vi "Process Injection Event Data.vi"(8 "error in (no error)":errorcluster, 10 "Injection.Results":T1 {"Measurements"."Shots"."Results"."Off-Stage Min Volt" format="%#.6g"; "Measurements"."Shots"."Results"."Off-Stage Avg Volt" format="%#.6g"; "Measurements"."Shots"."Results"."Off-Stage Max Volt" format="%#.6g"; "Measurements"."Shots"."Results"."Total Stage Time (us)" format="%#.6g"; "Measurements"."Shots"."Results"."Off-Stage Avg Current" format="%#.6g"; "Measurements"."Shots"."Results"."Total Voltage Pulses" format="%#.6g"; "Measurements"."Shots"."Results"."Off-Stage Min Current" format="%#.6g"; "Measurements"."Shots"."Results"."Off-Stage Max Current" format="%#.6g"}, 11 "Parameters":T4) -> (0 "error out":errorcluster, 3 "Parameters":T4)   [LabVIEW 2019, in "Fuel Injector Analysis Addon Engine.lvlib"]
uses:
  Fuel Injector Analysis Addon Engine.lvlib
  Types/Async Parameters.ctl
  Addon Shared/Types/Shot.Parameters.ctl
  Addon Shared/Types/Stage.Parameters.ctl
  Addon Shared/Types/Stage.PullIn.Types.ctl
  Addon Shared/Types/Stage.Transition.Types.ctl
  Addon Shared/Types/Analysis.Channels.Select.ctl
  Addon Shared/Types/Injector info.ctl
  Types/Injector.State.ctl
  <vilib>/NI/NIVS Inline Async API/_Data Access Engine/Data Access Engine/Types/Write.DVR.ctl
  <vilib>/NI/NIVS Inline Async API/_Data Access Engine/Access Type Classes/Write/Write.lvclass
  <vilib>/NI/NIVS Inline Async API/_Data Access Engine/Data Access Engine/Types/Read.DVR.ctl
  <vilib>/NI/NIVS Inline Async API/_Data Access Engine/Access Type Classes/Read/Read.lvclass
  Addon Shared/Types/Compiled.Group.WaveformRefs.ctl
  <vilib>/NI VeriStand/Custom Device API/Waveform Data Reference.ctl
  <vilib>/NI VeriStand/Custom Device Waveform API/Single Waveform Write (DBL)/Single Waveform Write (DBL).lvclass
  C:/Program Files (x86)/National Instruments/LabVIEW 2019/vi.lib/NI VeriStand/Custom Device Waveform API/Waveform Session.lvclass
  Types/Injector Event Data Cluster.ctl
  Types/Shot Information Control.ctl
  Types/Stage.Measurements.ctl
  <vilib>/NI/NIVS Inline Async API/_Data Access Engine/Access Type Classes/Read/Read.lvclass/Read.ctl
  <vilib>/NI VeriStand/Custom Device Waveform API/Waveform Session.lvclass/Waveform Session.ctl
  <vilib>/NI VeriStand/Custom Device Waveform API/Single Waveform Write (DBL)/Single Waveform Write (DBL).lvclass/Single Waveform Write (DBL).ctl
  <vilib>/NI VeriStand/Custom Device Waveform API/Internal Comm Classes/WPL Comm/WPL Comm (1D DBL)/WPL Comm (1D DBL).lvclass/WPL Comm (1D DBL).ctl
  <vilib>/NI VeriStand/Custom Device Waveform API/Internal Comm Classes/WPL Comm/WPL Comm.lvclass/WPL Comm.ctl
  <vilib>/NI/NIVS Inline Async API/_Data Access Engine/Access Type Classes/Write/Write.lvclass/Write.ctl
  <vilib>/NI VeriStand/Custom Device Waveform API/NI VeriStand - Write Waveform(s).vi
  <vilib>/NI VeriStand/Custom Device Waveform API/Single Waveform Write (DBL)/NI VeriStand - Write Single Waveform (DBL).vi
  <vilib>/NI/NIVS Inline Async API/_Data Access Engine/Data Access Engine/Methods/Data.Processes.Execute.vi
  <vilib>/NI/NIVS Inline Async API/_Data Access Engine/Data Access Engine/Methods/Read.Data.vi
  Build Result Array from Shots.vi
  <vilib>/NI/NIVS Inline Async API/_Data Access Engine/Data Access Engine/Methods/Write.Data.vi
  Calculate Current Magnitude Measurements.vi
  RT.Stages.Find.vi
  <vilib>/NI VeriStand/Custom Device Waveform API/Internal Comm Classes/WPL Comm/WPL Comm (1D DBL)/Comm_write 1d dbl.vi
  <vilib>/NI VeriStand/Custom Device Waveform API/Read Sample offset DVR.vi
  <vilib>/NI VeriStand/Custom Device Waveform API/Check Opened.vi
  <vilib>/NI/NIVS Inline Async API/_Data Access Engine/Access Type Classes/Read/Read.ProcessData.vi
  <vilib>/NI/NIVS Inline Async API/_Data Access Engine/Access Type Classes/Write/Write.ProcessData.vi
  Calculate Hold-In Measurements.vi
  <vilib>/Analysis/baseanly.llb/Mean.vi
  <vilib>/Analysis/baseanly.llb/Mean (DBL).vi
  Calculate Voltage Pulses.vi
  Calculate Hold-In Voltage Measurements.vi
  <vilib>/NI VeriStand/Custom Device Waveform API/Internal Comm Classes/WPL Comm/Direct Send WPL Command.vi
  <vilib>/NI VeriStand/Custom Device Waveform API/Internal Comm Classes/WPL Comm/Convert Q Error to Shutdown Error.vi
  <vilib>/NI/NIVS Inline Async API/_Data Access Engine/Access Type Classes/Write/Write.Buffer.vi
  <vilib>/NI/NIVS Inline Async API/_Data Access Engine/Access Type Classes/Write/Write.Commit.vi
  <vilib>/NI VeriStand/Custom Device Waveform API/Internal Comm Classes/WPL Comm/WPL Comm (1D DBL)/WPL Comm (1D DBL).lvclass
  C:/Program Files (x86)/National Instruments/LabVIEW 2019/vi.lib/NI VeriStand/Custom Device Waveform API/Internal Comm Classes/WPL Comm/WPL Comm.lvclass
  Addon Shared/SubVIs/Constants.vi
  <vilib>/Utility/error.llb/Error Cluster From Error Code.vi
  Addon Shared/Fuel Injector Analysis Addon Shared.lvlib
  <vilib>/NI VeriStand/Custom Device API/Custom Device API.lvlib
  <vilib>/NI/NIVS Inline Async API/_Data Access Engine/Data Access Engine/Data Access Engine.lvclass
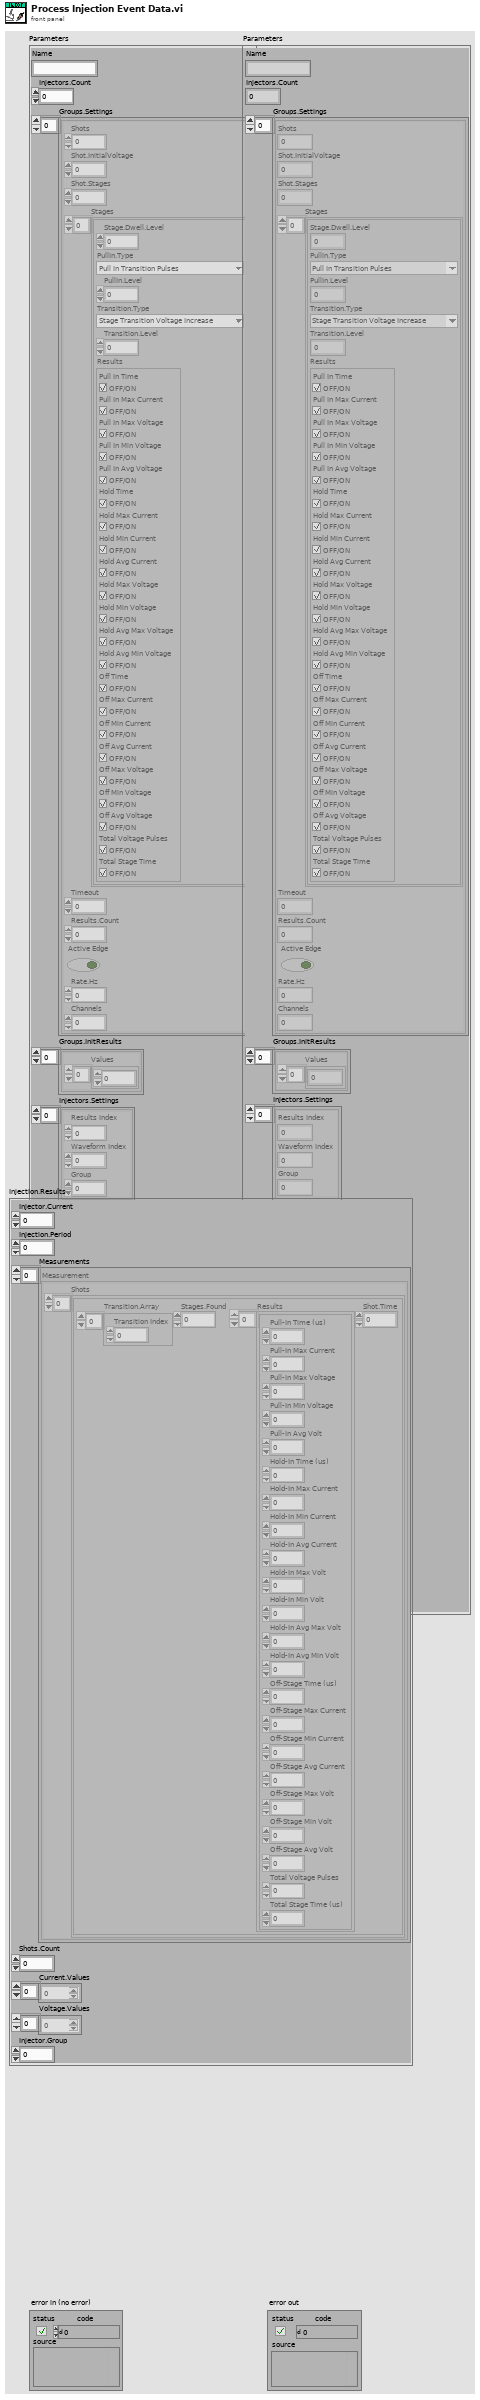
[diagram p1: front panel]
types:
  T1 = typedef "Fuel Injector Analysis Addon Engine.lvlib/Injector Event Data Cluster.ctl" = cluster{"Injector.Current":i16, "Injection.Period":dbl, "Measurements":cluster{"Shots":T2[]}[], "Shots.Count":i32, "Current.Values":dbl[], "Voltage.Values":dbl[], "Injector.Group":i16}
  T2 = typedef "Fuel Injector Analysis Addon Engine.lvlib/Shot Information Control.ctl" = cluster{"Transition.Array":i32[], "Stages.Found":u16, "Results":T3[], "Shot.Time":dbl}
  T3 = typedef "Fuel Injector Analysis Addon Engine.lvlib/Stage.Measurements.ctl" = cluster{"Pull-In Time (us)":dbl, "Pull-In Max Current":dbl, "Pull-In Max Voltage":dbl, "Pull-In Min Voltage":dbl, "Pull-In Avg Volt":dbl, "Hold-In Time (us)":dbl, "Hold-In Max Current":dbl, "Hold-In Min Current":dbl, "Hold-In Avg Current":dbl, "Hold-In Max Volt":dbl, "Hold-In Min Volt":dbl, "Hold-In Avg Max Volt":dbl, "Hold-In Avg Min Volt":dbl, "Off-Stage Time (us)":dbl, "Off-Stage Max Current":dbl, "Off-Stage Min Current":dbl, "Off-Stage Avg Current":dbl, "Off-Stage Max Volt":dbl, "Off-Stage Min Volt":dbl, "Off-Stage Avg Volt":dbl, "Total Voltage Pulses":dbl, "Total Stage Time (us)":dbl}
  T4 = typedef "Fuel Injector Analysis Addon Engine.lvlib/Async Parameters.ctl" = cluster{"Name":string, "Injectors.Count":u8, "Groups.Settings":T5[], "Groups.InitResults":cluster{"Values":dbl[]}[], "Injectors.Settings":T10[], "Injectors.State":T11[], "DMA.Ref":refnum<k20>, "FPGA.Status":T12, "Search.Data":T13, "Results.Data":T12, "Waveform.Enable":T13, "Waveform.Refs":T14[], "Waveform.Sessions":refnum<class "Single Waveform Write (DBL).lvclass">[]}
  T5 = typedef "Fuel Injector Analysis Addon Shared.lvlib/Shot.Parameters.ctl" = cluster{"Shots":u32, "Shot.InitialVoltage":dbl, "Shot.Stages":u32, "Stages":T6[], "Timeout":dbl, "Results.Count":i32, "Active Edge":bool, "Rate.Hz":u32, "Channels":u32}
  T6 = typedef "Fuel Injector Analysis Addon Shared.lvlib/Stage.Parameters.ctl" = cluster{"Stage.Dwell.Level":dbl, "PullIn.Type":T7, "PullIn.Level":dbl, "Transition.Type":T8, "Transition.Level":dbl, "Results":T9}
  T7 = typedef "Fuel Injector Analysis Addon Shared.lvlib/Stage.PullIn.Types.ctl" = enum8{"Pull In Transition Pulses", "Pull In Transition Current Drop"}
  T8 = typedef "Fuel Injector Analysis Addon Shared.lvlib/Stage.Transition.Types.ctl" = enum8{"Stage Transition Inactive Time", "Stage Transition Voltage Increase", "Stage Transition Current Decrease", "Stage Transition Active Time"}
  T9 = typedef "Fuel Injector Analysis Addon Shared.lvlib/Analysis.Channels.Select.ctl" = cluster{"Pull In Time":bool, "Pull In Max Current":bool, "Pull In Max Voltage":bool, "Pull In Min Voltage":bool, "Pull In Avg Voltage":bool, "Hold Time":bool, "Hold Max Current":bool, "Hold Min Current":bool, "Hold Avg Current":bool, "Hold Max Voltage":bool, "Hold Min Voltage":bool, "Hold Avg Max Voltage":bool, "Hold Avg Min Voltage":bool, "Off Time":bool, "Off Max Current":bool, "Off Min Current":bool, "Off Avg Current":bool, "Off Max Voltage":bool, "Off Min Voltage":bool, "Off Avg Voltage":bool, "Total Voltage Pulses":bool, "Total Stage Time":bool}
  T10 = typedef "Fuel Injector Analysis Addon Shared.lvlib/Injector info.ctl" = cluster{"Results Index":i32, "Waveform Index":i32, "Group":u16}
  T11 = typedef "Fuel Injector Analysis Addon Engine.lvlib/Injector.State.ctl" = cluster{"Timer":u32, "Events":u64}
  T12 = typedef "Data Access Engine.lvlib/Data Access Engine.lvclass/Write.DVR.ctl" = refnum<data-value>
  T13 = typedef "Data Access Engine.lvlib/Data Access Engine.lvclass/Read.DVR.ctl" = refnum<data-value>
  T14 = typedef "Fuel Injector Analysis Addon Shared.lvlib/Compiled.Group.WaveformRefs.ctl" = cluster{"WaveformRefs":T15[], "Group":i32}
  T15 = typedef "Custom Device API.lvlib/Waveform Data Reference.ctl" = i32
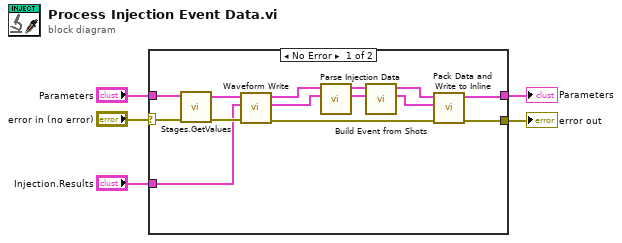
[diagram p0: block diagram]
diagram:
  n1 = case shown="No Error" "error in (no error)" {
    selector: "error in (no error)" -> [w17 w21]
    tunnel: "Parameters" -> [w15 w20]
    tunnel: [w19 w21] -> w3
    tunnel: [w6 w20] -> w2
    tunnel: "Injection.Results" -> [w13 _]
    frame No Error {
      n2 = call "Stages.GetValues.vi"("error in (no error)"=w17, "Async Parameters in"=w15) -> ("error out"=w16:errorcluster, "Async Parameters out"=w14:T4)  [unwired: 8 in]
      n3 = call "Waveform Write.vi"("error in (no error)"=w16, "Injection.Results"=w13, "Parameters"=w14) -> ("error out"=w18:errorcluster, "Injection.Results"=w11:T1, "Parameters"=w12:T4)  [unwired: 6 in]
      n4 = call "Parse Injection Data.vi"("Injection.Results"=w11, "Parameters"=w12) -> ("Injection.Results"=w7:T1, "Parameters"=w8:T4)  [unwired: 8 in]
      n5 = call "Build Event from Shots.vi"("Injection.Results"=w7, "Parameters"=w8) -> ("Injection.Results"=w10:T1, "Parameters"=w9:T4)  [unwired: 8 in]
      n6 = call "Pack Data and Write to Inline.vi"("Error In"=w18, "Injection Event Data Cluster"=w10, "Async Parameters"=w9) -> ("Error out"=w19:errorcluster, "Async Parameters out"=w6:T4)  [unwired: 7 in]
    }
    frame Error {
    }
  }
  "error out" <- w3
  "Parameters" <- w2
